vi "Untitled 1.vi"() -> ()   [LabVIEW 2017]
panel:
  out "Variant cluster":T1
  out "# elements in queue":i32
  out "TempsLabels":T2(array[cluster])
  in  "array":variant[](array[variant])
  in  "Cluster":T3
  out "TempData":bool=TRUE
  in  "temp typedef":dbl[][](array[numeric])
  in  "Array 5":dbl[][](array[numeric])
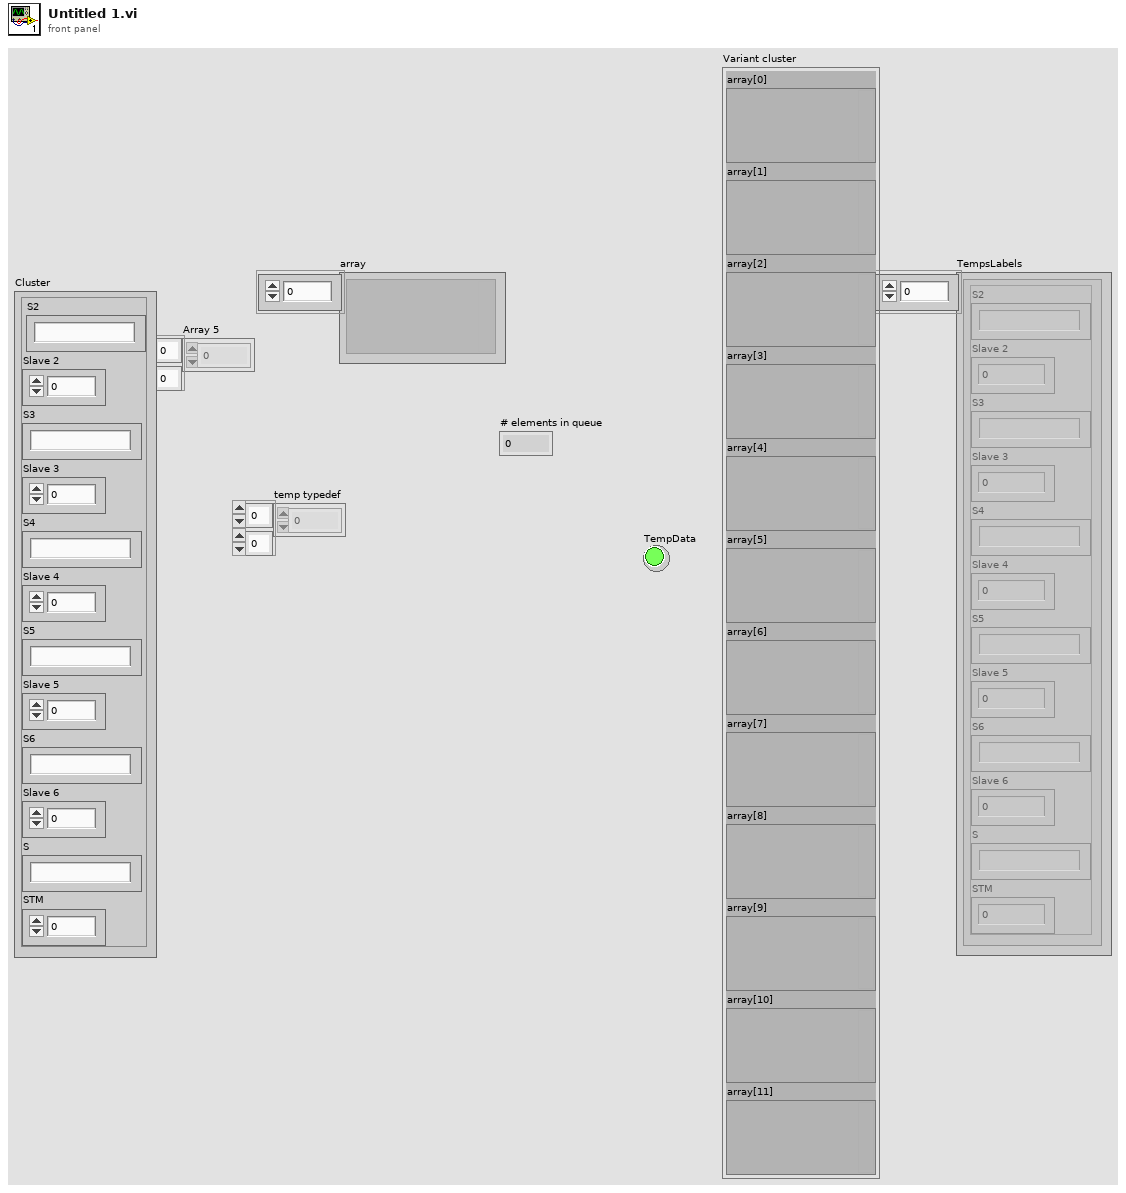
[diagram p1: front panel]
types:
  T1 = cluster{"array[0]":variant, "array[1]":variant, "array[2]":variant, "array[3]":variant, "array[4]":variant, "array[5]":variant, "array[6]":variant, "array[7]":variant, "array[8]":variant, "array[9]":variant, "array[10]":variant, "array[11]":variant}
  T2 = cluster{"S2":string, "Slave 2":dbl, "S3":string, "Slave 3":dbl, "S4":string, "Slave 4":dbl, "S5":string, "Slave 5":dbl, "S6":string, "Slave 6":dbl, "S":string, "STM":dbl}[]
  T3 = cluster{"S2":string, "Slave 2":dbl, "S3":string, "Slave 3":dbl, "S4":string, "Slave 4":dbl, "S5":string, "Slave 5":dbl, "S6":string, "Slave 6":dbl, "S":string, "STM":dbl}
  T4 = cluster{"Termometr 1":string, "Termometr 2":string, "Termometr 3":string, "Termometr 4":string, "Termometr 5":string, "Termometr 6":string, "Termometr 7":string, "Termometr 8":string, "Termometr 9":string, "Termometr 10":string}
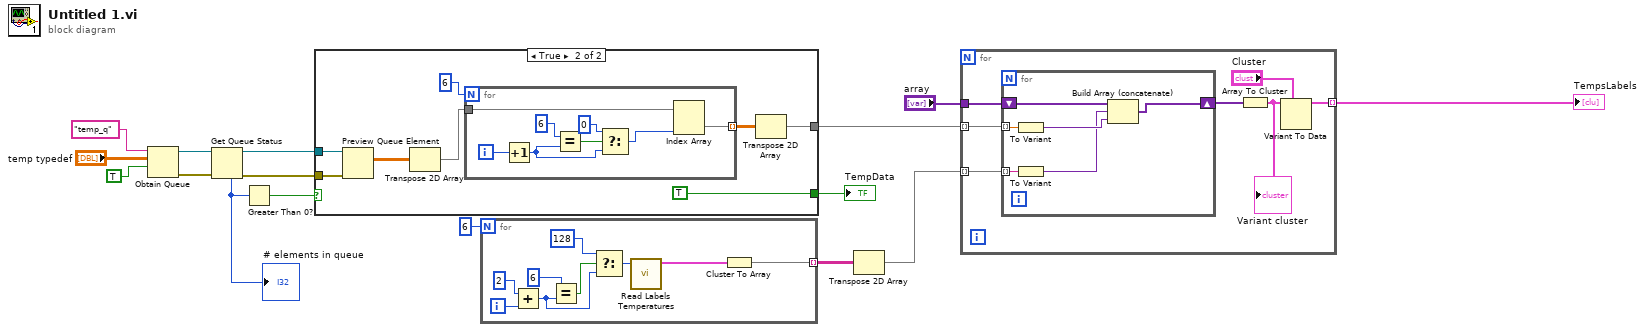
[diagram p0: block diagram]
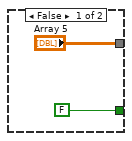
[diagram p2: hidden frame]
diagram:
  n1 = Obtain Queue(name (unnamed)="temp_q", element data type="temp typedef", create if not found? (T)=TRUE) -> (queue out=w8:refnum<queue>, error out=w9:errorcluster)  [unwired: 2 in, 1 out]
  n2 = Get Queue Status(queue=w8, error in (no error)=w9) -> (queue out=w14:refnum<queue>, error out=w15:errorcluster, # elements in queue=w16:i32)  [unwired: 1 in, 5 out]
  "# elements in queue" <- w16
  n3 = Greater Than 0?(x=w16) -> (x > 0?=w13:bool)
  n4 = case shown="True" w13 {
    tunnel: w15 -> [_ w25]
    tunnel: w14 -> [_ w26]
    tunnel: ["Array 5" w19] -> w4
    tunnel: [FALSE TRUE] -> w7
    frame False {
    }
    frame True {
      n5 = Preview Queue Element(queue=w26, error in (no error)=w25) -> (element=w23:dbl[][])  [unwired: 1 in, 3 out]
      n6 = Transpose 2D Array(2D array=w23) -> (transposed array=w21:dbl[][])
      n7 = for {
        N: 6 -> [_]
        tunnel: w21 -> [w33]
        tunnel: [w32] -> w20 mode=indexing
        i -> [w34]
        n8 = Increment(x=w34) -> (x+1=w27:i32)
        n9 = Equal?(x=6 ("y"), y=w27) -> (x = y?=w31:bool)
        n10 = Select(t=0, s=w31, f=w27) -> (s? t:f=w28:i32)
        n11 = Index Array(array=w33, index (col)=w28) -> (element=w32:dbl[])  [unwired: 1 in]
      }
      n12 = Transpose 2D Array(2D array=w20) -> (transposed array=w19:dbl[][])
    }
  }
  "TempData" <- w7
  n13 = for {
    N: 6 -> [_]
    tunnel: [w35] -> w5 mode=indexing
    i -> [w43]
    n14 = Add(x=2, y=w43) -> (x+y=w38:i32)
    n15 = Equal?(x=6, y=w38) -> (x = y?=w39:bool)
    n16 = Select(t=128, s=w39, f=w38) -> (s? t:f=w41:i32)
    n17 = call "Read Labels Temperatures.vi"("Slave ID"=w41) -> ("Etykiety T1-10"=w36:T4)  [unwired: 10 in]
    n18 = Cluster To Array(cluster=w36) -> (array=w35:string[])
  }
  n19 = Transpose 2D Array(2D array=w5) -> (transposed array=w3:string[][])
  n20 = for {
    tunnel: w4 -> [w49] mode=indexing
    tunnel: w3 -> [w50] mode=indexing
    tunnel: "array" -> [w48]
    tunnel: [w44] -> w1 mode=indexing
    n21 = for {
      tunnel: w50 -> [w55] mode=indexing
      tunnel: w49 -> [w56] mode=indexing
      shift-right: [w53] -> w47
      shift-left: w48 -> [w54]
      n22 = To Variant(anything=w56) -> (Variant=w52:variant)
      n23 = To Variant(anything=w55) -> (Variant=w51:variant)
      n24 = Build Array (concatenate)(w54, w51, w52) -> (w53:variant[])
    }
    n25 = Array To Cluster(array=w47) -> (cluster=w46:T1)
    "Variant cluster" <- w46
    n26 = Variant To Data(type="Cluster", Variant=w46) -> (data=w44:T3)  [unwired: 1 in, 1 out]
  }
  "TempsLabels" <- w1
